vi "use designated z spacing (SubVI).vi"(2 "use designated z spacing":bool=TRUE, 3 "file path":path) -> (1 "path":path)   [LabVIEW 2024]
uses:
  Global variables/global for picoscope.vi
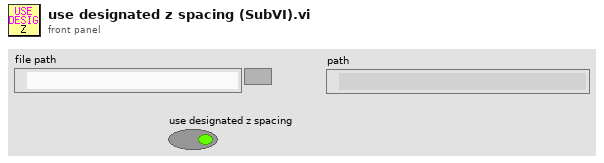
[diagram p1: front panel]
types:
  T1 = enum16{"open", "replace", "create", "open or create", "replace or create", "replace or create with confirmation"}
  T2 = cluster{"img scan pos":dbl[][], "g1 disp [um]":dbl, "z spacing [um]":dbl, "g2 disp [pixels]":dbl, "scape scan pos ":dbl[]}
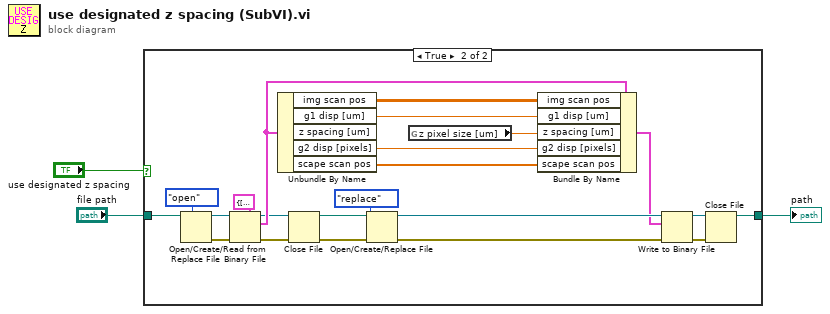
[diagram p0: block diagram]
diagram:
  n1 = case shown="True" "use designated z spacing" {
    tunnel: "file path" -> [w4 w7]
    tunnel: [w4 w6] -> w2
    frame False {
    }
    frame True {
      n2 = Open/Create/Replace File(file path (use dialog)=w7, operation (0:open)=T1."open") -> (refnum out=w25:refnum<file>, error out=w24:errorcluster)  [unwired: 4 in, 1 out]
      n3 = Read from Binary File(5:T2 {"img scan pos"=[], "g1 disp [um]"=0.0, "z spacing [um]"=0.0, "g2 disp [pixels]"=0.0, "scape scan pos "=[]} ("output cluster 2"), 8:w24, 11:w25) -> (0:w14:errorcluster, 2:w23:T2, 3:w15:refnum<file>)  [unwired: 3 in, 1 out]
      n4 = Unbundle By Name(w23) -> ("img scan pos"=w22:dbl[][], "g1 disp [um]"=w21:dbl, "g2 disp [pixels]"=w20:dbl, "scape scan pos"=w19:dbl[])  [unwired: 1 out]
      n5 = Close File(refnum=w15, error in=w14) -> (path=w13:path, error out=w12:errorcluster)
      n6 = Open/Create/Replace File(file path (use dialog)=w13, error in=w12, operation (0:open)=T1."replace") -> (refnum out=w11:refnum<file>, error out=w10:errorcluster)  [unwired: 3 in, 1 out]
      n7 = global read "global for picoscope.vi" "z pixel size [um]"() -> (w5:dbl)
      n8 = Bundle By Name(cluster=w23, "img scan pos"=w22, "g1 disp [um]"=w21, "z spacing [um]"=w5, "g2 disp [pixels]"=w20, "scape scan pos"=w19) -> (w9:T2)
      n9 = Write to Binary File(file (use dialog)=w11, data=w9, error in=w10) -> (refnum out=w18:refnum<file>, error out=w17:errorcluster)  [unwired: 3 in, 1 out]
      n10 = Close File(refnum=w18, error in=w17) -> (path=w6:path)  [unwired: 1 out]
    }
  }
  "path" <- w2
